vi "MeasurementServer_SetResponse_Config.vi"(0 "gRPCid":T1, 1 "acknowledge":bool, 3 "error in (no error)":errorcluster) -> (10 "error out":errorcluster)   [LabVIEW 2019, in "labview-grpc-measurement-server.lvlib"]
uses:
  labview-grpc-measurement-server.lvlib
  MeasurementServer_gRPCid.ctl
  home/lvuser/liblabview_measurement_server.so
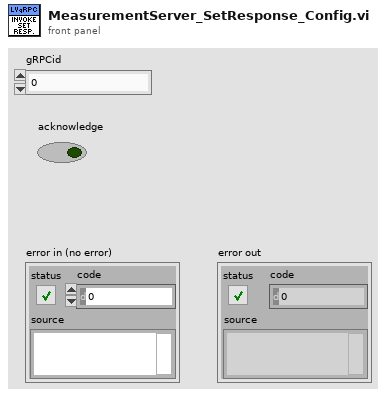
[diagram p1: front panel]
types:
  T1 = typedef "labview-grpc-measurement-server.lvlib/MeasurementServer_gRPCid.ctl" = u64
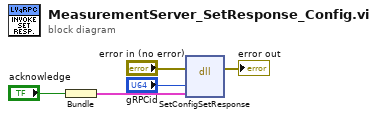
[diagram p0: block diagram]
diagram:
  n1 = Bundle("acknowledge"="acknowledge") -> (w2:cluster{"acknowledge":bool})  [unwired: 1 in]
  n2 = dll-call lib="home/lvuser/liblabview_measurement_server.so" fn="SetConfigSetResponse"(error in="error in (no error)", "id"="gRPCid", "data"=w2) -> (error out=→"error out":errorcluster)  [unwired: 5 in, 1 out]
